vi "Store Session Info to Unreserve.vi"(8 "error in":errorcluster, 10 "session reservation":refnum<class "Session Reservation.lvclass">, 11 "measurement context in":refnum<class "MeasurementContext.lvclass">) -> (0 "error out":errorcluster, 3 "measurement context out":refnum<class "MeasurementContext.lvclass">)   [LabVIEW 2020, in "MeasurementLink Measurement Server.lvlib" / "MeasurementContext.lvclass"]
uses:
  MeasurementContext.lvclass
  MeasurementContext.lvclass/MeasurementContext.ctl
  MeasurementLink Session Management/Session Reservation/Session Reservation.lvclass
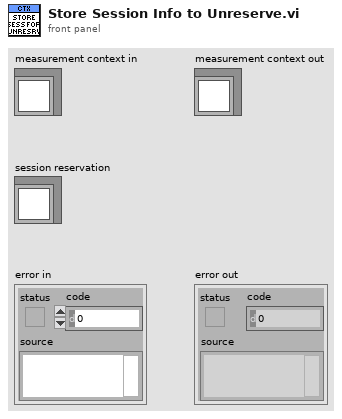
[diagram p1: front panel]
types:
  T1 = typedef "MeasurementLink Measurement Server.lvlib/MeasurementContext.lvclass/Data.ctl" = cluster{"PinMapContext":T2, "gRPCServerId":T3, "IMeasurementService":refnum<class "IMeasurementService.lvclass">, "MeasurementPluginService":refnum<class "MeasurementPluginService.lvclass">, "session infos to unreserve":map{refnum<class "Session Reservation.lvclass">, T4[]}}
  T2 = typedef "MeasurementLink Measurement Server.lvlib/PinMapContext.ctl" = cluster{"pin_map_id":string, "sites":i32[]}
  T3 = typedef "grpc-lvsupport-release.lvlib/grpcId.ctl" = u64
  T4 = typedef "MeasurementLink Session Management Client.lvlib/ni_measurementlink_sessionmanagement_v1_SessionInformation.ctl" = cluster{"session":T5, "resource_name":string, "channel_list":string, "instrument_type_id":string, "session_exists":bool, "channel_mappings":T6[]}
  T5 = typedef "MeasurementLink Session Management Client.lvlib/nidevice_grpc_Session.ctl" = cluster{"name":string}
  T6 = typedef "MeasurementLink Session Management Client.lvlib/ni_measurementlink_sessionmanagement_v1_ChannelMapping.ctl" = cluster{"pin_or_relay_name":string, "site":i32, "channel":string}
  T7 = map{refnum<class "Session Reservation.lvclass">, T4[]}
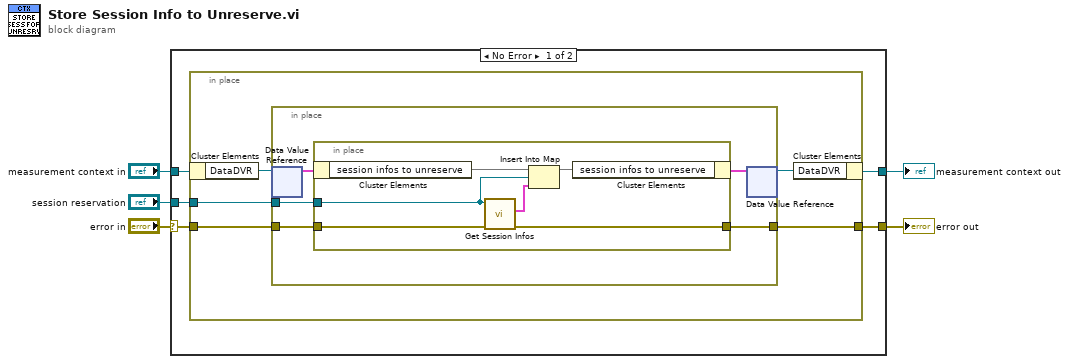
[diagram p0: block diagram]
diagram:
  n1 = case shown="No Error" "error in" {
    selector: "error in" -> [w7 w28]
    tunnel: [w6 w28] -> w4
    tunnel: [w9 w27] -> w2
    tunnel: "measurement context in" -> [w10 w27]
    tunnel: "session reservation" -> [w8 _]
    frame No Error {
      n2 = in-place {
        in-place-border: w8 -> [w13]
        in-place-border: w7 -> [w12]
        in-place-border: [w11] -> w6
        n3 = in-place-cluster #1(w10) -> ("DataDVR"=w15:refnum<data-value>)
        n4 = in-place {
          in-place-border: w13 -> [w18]
          in-place-border: w12 -> [w17]
          in-place-border: [w16] -> w11
          n5 = in-place-dvr #2(w15) -> (w20:T1)  [unwired: 1 out]
          n6 = in-place {
            in-place-border: w18 -> [w22]
            in-place-border: w17 -> [w26]
            in-place-border: [w25] -> w16
            n7 = in-place-cluster #3(w20) -> ("session infos to unreserve"=w23:T7)
            n8 = call "Get Session Infos.vi"("error in"=w26, "session reservation in"=w22) -> ("error out"=w25:errorcluster, "session infos"=w24:T4[])  [unwired: 7 in, 1 out]
            n9 = Insert Into Map(map in=w23, key=w22, value=w24) -> (map out=w21:T7)  [unwired: 2 out]
            n10 = in-place-cluster #3("session infos to unreserve"=w21) -> (w19:T1)
          }
          n11 = in-place-dvr #2(w19) -> (w14:refnum<data-value>)  [unwired: 1 out]
        }
        n12 = in-place-cluster #1("DataDVR"=w14) -> (w9:refnum<class "MeasurementContext.lvclass">)
      }
    }
    frame Error {
    }
  }
  "error out" <- w4
  "measurement context out" <- w2
